vi "Set Overpressure Strategy.vi"(8 "error in (no error)":errorcluster, 11 "ASIA Pump # In":i32) -> (0 "error out":errorcluster, 2 "strategySet":bool, 3 "ASIA Pump # Out":i32)   [LabVIEW 2018, in "ASIA Pump.lvlib"]
uses:
  ASIA Pump.lvlib
panel:
  out "path out":path
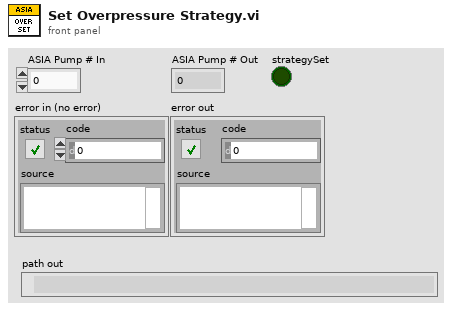
[diagram p1: front panel]
types:
  T1 = cluster{"Busy":bool, "PumpCnt":dbl, "RemoteEntered":bool, "OverpressureSet":bool}[]
  T2 = cluster{"Busy":bool, "PumpCnt":dbl, "RemoteEntered":bool, "OverpressureSet":bool}
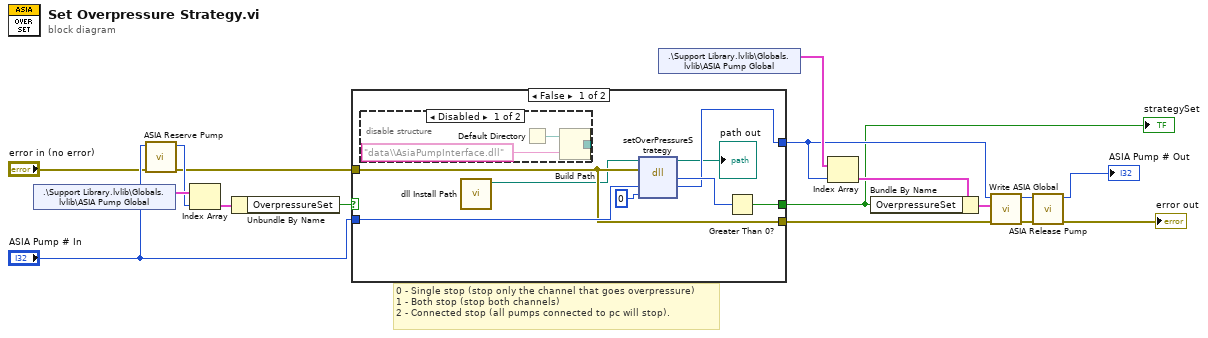
[diagram p0: block diagram]
diagram:
  # "0 - Single stop (stop only the channel that goes overpressure)\n1 - Both stop (stop both channels)\n2 - Connected stop (all pumps connected to pc will stop)."
  n1 = shared-variable ".\\Support Library.lvlib\\Globals.lvlib\\ASIA Pump Global"() -> (w17:T1)  [unwired: 1 in, 1 out]
  n2 = call "ASIA Reserve Pump.vi"("error in (no error)"="error in (no error)", "ASIA Pump # In"="ASIA Pump # In") -> ("error out"=w11:errorcluster, "ASIA Pump # Out"=w13:i32)  [unwired: 8 in]
  n3 = Index Array(array=w17, index=w13) -> (element=w16:T2)
  n4 = Unbundle By Name(w16) -> ("OverpressureSet"=w15:bool)
  n5 = case shown="False" w15 {
    selector: w15 -> [_ w31]
    tunnel: w11 -> [w20 w29]
    tunnel: "ASIA Pump # In" -> [w24 w30]
    tunnel: [w22 w31] -> w6
    tunnel: [w21 w30] -> w7
    tunnel: [w20 w29] -> w8
    frame False {
      n6 = disable-structure shown="Disabled" {
        disable-tunnel: [w26 _] -> _
        frame Disabled {
          n7 = Default Directory() -> (w27:path)
          n8 = Build Path(base path=w27, name or relative path="data\\AsiaPumpInterface.dll") -> (appended path=w26:path)
        }
        frame Enabled {
        }
      }
      n9 = call "dll Install Path.vi"() -> ("system directory"=w19:path)  [unwired: 11 in]
      n10 = dll-call lib="C:/Program Files (x86)/Pfizer/FAST/data/AsiaPumpInterface.dll" fn="setOverPressureStrategy"(path in=w19, error in=w20, "pumpNum"=w24, "strategy"=u8 0) -> (path out=→"path out":path, "Bool"=w23:u8, "pumpNum"=w21:u32)  [unwired: 2 in, 1 out]
      n11 = Greater Than 0?(x=w23) -> (x > 0?=w22:bool)
    }
    frame True {
    }
  }
  "strategySet" <- w6
  n12 = shared-variable ".\\Support Library.lvlib\\Globals.lvlib\\ASIA Pump Global"() -> (w9:T1)  [unwired: 1 in, 1 out]
  n13 = Index Array(array=w9, index=w7) -> (element=w10:T2)
  n14 = Bundle By Name(cluster=w10, "OverpressureSet"=w6) -> (w5:T2)
  n15 = call "Write ASIA Global.vi"("error in (no error)"=w8, "ASIA Global"=w5, "Pump Number In"=w7) -> ("error out"=w2:errorcluster, "Pump Number Out"=w4:i32)  [unwired: 7 in]
  n16 = call "ASIA Release Pump.vi"("error in (no error)"=w2, "pumpNum"=w4) -> ("error out"=→"error out":errorcluster, "ASIA Pump # Out"=→"ASIA Pump # Out":i32)  [unwired: 8 in]
